vi "fill the pulse memory_12 memors.vi"(10 "memory units":T1={"Memory In"="pulse on memory", "Memory In 2"="", "Memory In 3"="", "Memory In 6"="pulse on memory", "Memory In 4"="pulse on memory", "Memory In 5"="", "Memory In 7"="", "Memory In 8"="pulse on memory", "Memory In 9"="pulse on memory", "Memory In 10"="", "Memory In 11"="", "Memory In 12"="pulse on memory"}, 11 "FIFO In":refnum<k21>="fifo pulse from host") -> ()   [LabVIEW 2021]
uses:
  <vilib>/rvi/DataTransferAndStorage/Container/Common/niFpgaContainerExecOnDevCompGetState.vi
  <vilib>/rvi/Emulation/niFpgaEmulationIsFPGAContextNoSignature.vi
  <vilib>/rvi/DataTransferAndStorage/Container/Common/niFpgaContainerGetUniqueNameForEmu.vi
  <vilib>/rvi/Emulation/niFpgaProcessEmulError.vi
  <vilib>/rvi/Emulation/niFpgaSctlEmulationGetInTimedLoop.vi
  <vilib>/rvi/errors/nirviReportUnexpectedCaseInternalError (U32).vi
  <vilib>/rvi/Memory/Memory_Emulation/niFpgaMemoryEmulationCacheClearOnFirstRun.vi
  <vilib>/rvi/Memory/Memory_Emulation/nirvimemoryEmulationManagerCache_MakeExclusive.vi
  <vilib>/rvi/Memory/Memory_Emulation/niFpgaMemoryEmulationValidateCache.vi
  <vilib>/rvi/Memory/Memory_Emulation/nirvimemoryEmulationManagerCache_InsertValue.vi
  <vilib>/Utility/error.llb/Clear Errors.vi
  <vilib>/rvi/Memory/Memory_Emulation/nirvimemoryEmulationManagerCache_ReleaseExclusive.vi
  <vilib>/rvi/Memory/Memory_Emulation/nirvimemoryEmulationManagerCache_GetValue.vi
  <vilib>/rvi/Memory/Memory_Emulation/nirvimemoryEmulationManagerCache_SetValue.vi
  <vilib>/rvi/Emulation/niFpgaSctlEmulationResourceMgr.vi
  <vilib>/rvi/errors/niFpgaSetErrorForExecOnDevCompSimple.vi
  <vilib>/rvi/eio/common/nirviEmuReportErrorAndStop.vi
  <vilib>/rvi/FIFO/Fifo_Resource/nirvififoEmulationSetSize.vi
  <vilib>/rvi/FIFO/Fifo_Resource/nirviFifoEmulationQueueMgr.vi
  <instcachedir>/0/nirviFifoEmulationQueueMgr_E5CAEC123FF24DC58D834DCA3CDAA9B5.lvgen/nirviFifoEmulationQueueMgr_E5CAEC123FF24DC58D834DCA3CDAA9B5_008.vi
  <vilib>/rvi/FIFO/Fifo_Resource/nirvififoEmulationDetermineInputValidOut.vi
  <vilib>/rvi/FIFO/Fifo_Resource/nirvififoEmulationCreateLock.vi
  <vilib>/rvi/FIFO/Fifo_Resource/nirvififoEmulationObtainLock.vi
  <vilib>/rvi/FIFO/Fifo_Resource/nirvififoEmulationReleaseLock.vi
  <vilib>/rvi/occurrence/nirviWaitOnOccurrenceBase.vi
  <vilib>/rvi/errors/nirviReportUnexpectedCaseInternalError.vi
  <vilib>/rvi/interface/RandomDataEmulation/niFpgaRandomDataHandleErrors.vi
  <vilib>/rvi/DataTransferAndStorage/Container/XNode/niFpgaContainer.xnode
  <vilib>/rvi/Memory/Memory_Emulation/niFpgaMemoryEmulationRefIn.vi
  <vilib>/rvi/FIFO/Fifo_Resource/niFpgaFifoEmulationRefIn.vi
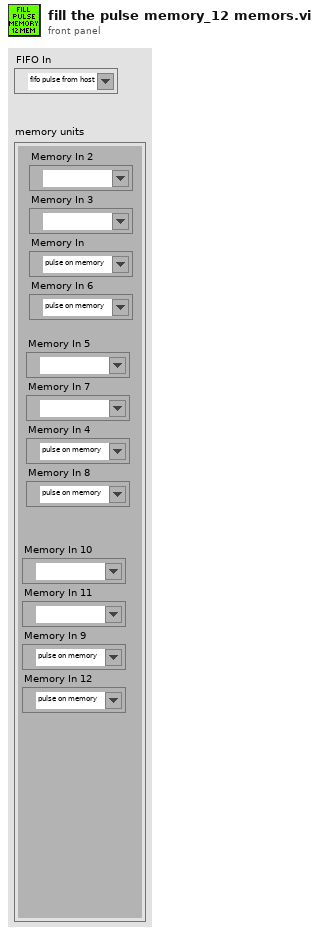
[diagram p1: front panel]
types:
  T1 = cluster{"Memory In":refnum<k21>, "Memory In 2":refnum<k21>, "Memory In 3":refnum<k21>, "Memory In 6":refnum<k21>, "Memory In 4":refnum<k21>, "Memory In 5":refnum<k21>, "Memory In 7":refnum<k21>, "Memory In 8":refnum<k21>, "Memory In 9":refnum<k21>, "Memory In 10":refnum<k21>, "Memory In 11":refnum<k21>, "Memory In 12":refnum<k21>}
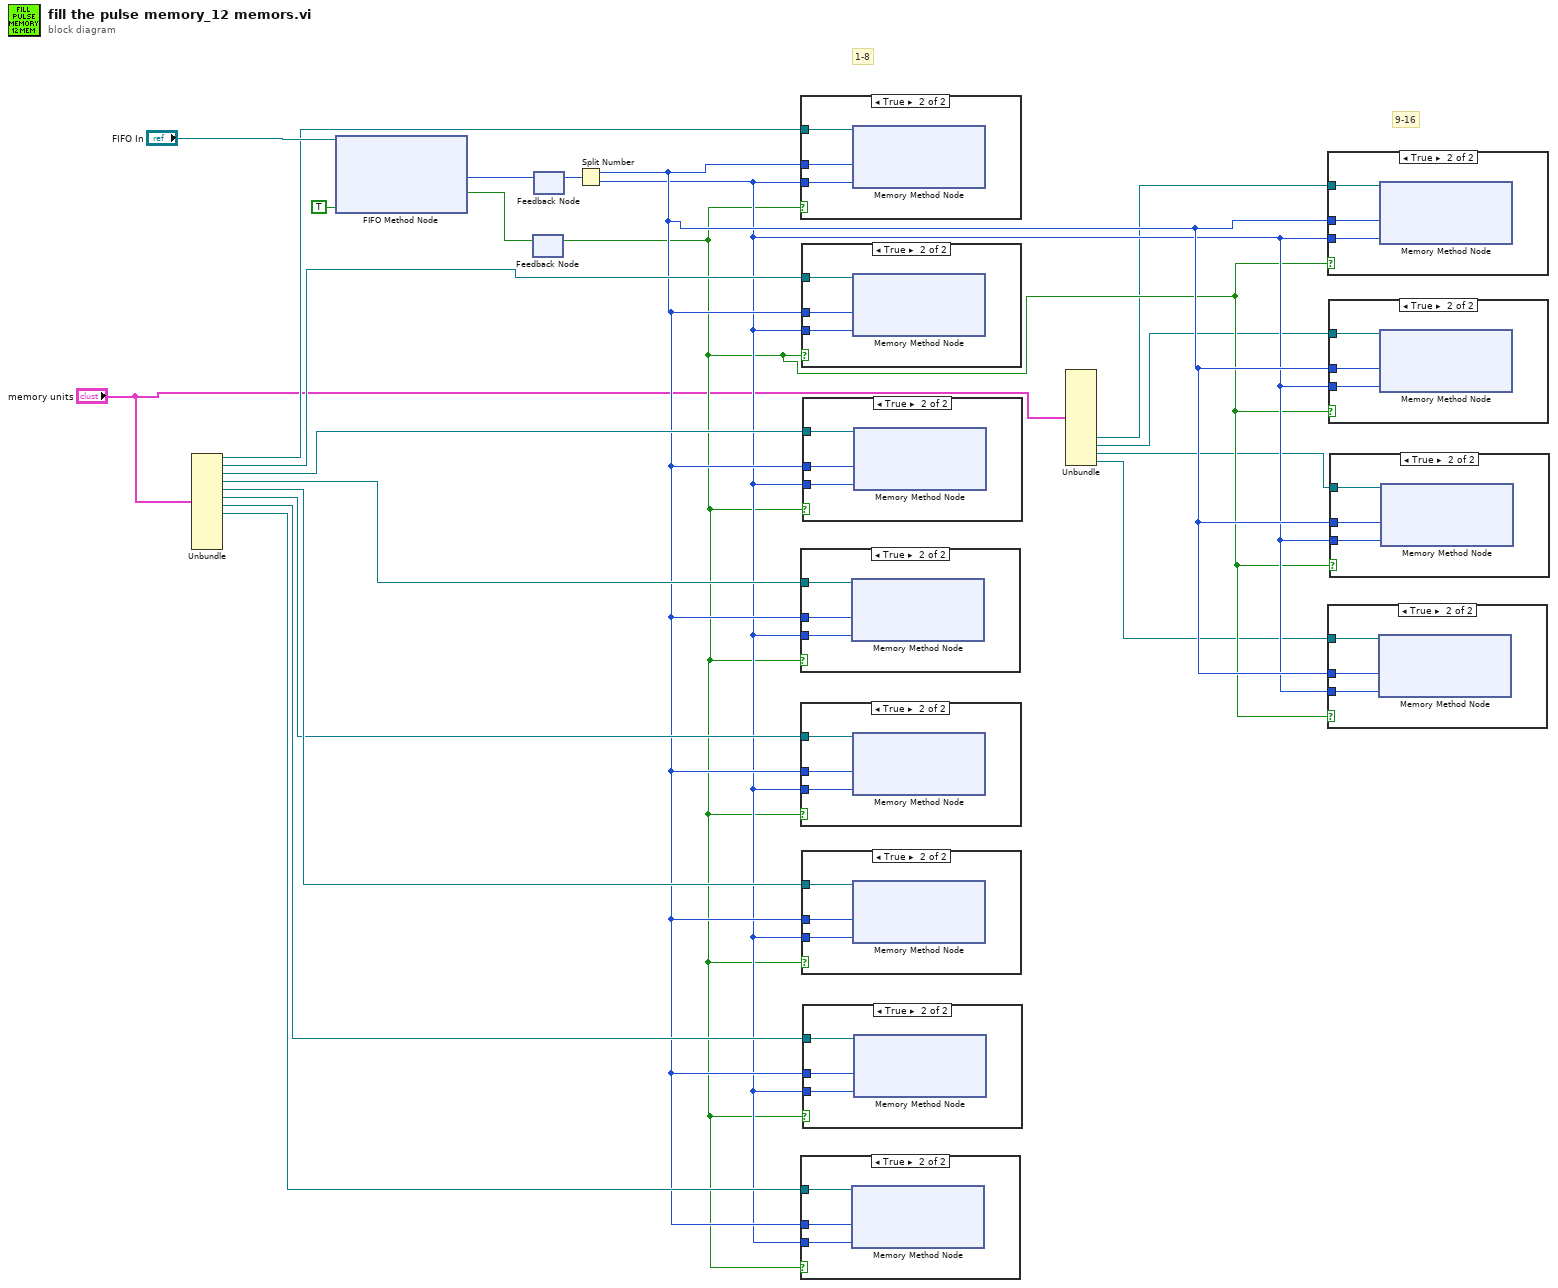
[diagram p0: block diagram]
diagram:
  # "9-16"
  # "1-8"
  n1 = Unbundle("memory units") -> ("Memory In"=w19:refnum<k21>, "Memory In 2"=w18:refnum<k21>, "Memory In 3"=w17:refnum<k21>, "Memory In 6"=w16:refnum<k21>, "Memory In 4"=w15:refnum<k21>, "Memory In 5"=w14:refnum<k21>, "Memory In 7"=w13:refnum<k21>, "Memory In 8"=w12:refnum<k21>)  [unwired: 4 out]
  n2 = xnode ("FIFO Method Node")("Ready for Output"=TRUE, "FIFO In"="FIFO In") -> ("Element"=w10:u64, "Output Valid"=w11:bool)  [unwired: 1 out]
  n3 = feedback-in #1(w11) -> ()
  n4 = feedback #1() -> (w6:bool)  [unwired: 1 in]
  n5 = feedback #2() -> (w9:u64)  [unwired: 1 in]
  n6 = feedback-in #2(w10) -> ()
  n7 = Split Number(x=w9) -> (hi(x)=w8:u32, lo(x)=w7:u32)
  n8 = case shown="True" w6 {
    tunnel: w8 -> [_ w24]
    tunnel: w7 -> [_ w23]
    tunnel: w19 -> [_ w22]
    frame False {
    }
    frame True {
      n9 = xnode ("Memory Method Node")("Address"=w24, "Data"=w23, "Memory In"=w22) -> ()  [unwired: 1 out]
    }
  }
  n10 = case shown="True" w6 {
    tunnel: w8 -> [_ w27]
    tunnel: w7 -> [_ w26]
    tunnel: w16 -> [_ w25]
    frame False {
    }
    frame True {
      n11 = xnode ("Memory Method Node")("Address"=w27, "Data"=w26, "Memory In"=w25) -> ()  [unwired: 1 out]
    }
  }
  n12 = case shown="True" w6 {
    tunnel: w8 -> [_ w30]
    tunnel: w7 -> [_ w29]
    tunnel: w14 -> [_ w28]
    frame False {
    }
    frame True {
      n13 = xnode ("Memory Method Node")("Address"=w30, "Data"=w29, "Memory In"=w28) -> ()  [unwired: 1 out]
    }
  }
  n14 = case shown="True" w6 {
    tunnel: w8 -> [_ w33]
    tunnel: w7 -> [_ w32]
    tunnel: w12 -> [_ w31]
    frame False {
    }
    frame True {
      n15 = xnode ("Memory Method Node")("Address"=w33, "Data"=w32, "Memory In"=w31) -> ()  [unwired: 1 out]
    }
  }
  n16 = case shown="True" w6 {
    tunnel: w8 -> [_ w36]
    tunnel: w7 -> [_ w35]
    tunnel: w18 -> [_ w34]
    frame False {
    }
    frame True {
      n17 = xnode ("Memory Method Node")("Address"=w36, "Data"=w35, "Memory In"=w34) -> ()  [unwired: 1 out]
    }
  }
  n18 = case shown="True" w6 {
    tunnel: w8 -> [_ w39]
    tunnel: w7 -> [_ w38]
    tunnel: w15 -> [_ w37]
    frame False {
    }
    frame True {
      n19 = xnode ("Memory Method Node")("Address"=w39, "Data"=w38, "Memory In"=w37) -> ()  [unwired: 1 out]
    }
  }
  n20 = case shown="True" w6 {
    tunnel: w8 -> [_ w42]
    tunnel: w7 -> [_ w41]
    tunnel: w17 -> [_ w40]
    frame False {
    }
    frame True {
      n21 = xnode ("Memory Method Node")("Address"=w42, "Data"=w41, "Memory In"=w40) -> ()  [unwired: 1 out]
    }
  }
  n22 = case shown="True" w6 {
    tunnel: w8 -> [_ w45]
    tunnel: w7 -> [_ w44]
    tunnel: w13 -> [_ w43]
    frame False {
    }
    frame True {
      n23 = xnode ("Memory Method Node")("Address"=w45, "Data"=w44, "Memory In"=w43) -> ()  [unwired: 1 out]
    }
  }
  n24 = Unbundle("memory units") -> ("Memory In 9"=w1:refnum<k21>, "Memory In 10"=w2:refnum<k21>, "Memory In 11"=w3:refnum<k21>, "Memory In 12"=w4:refnum<k21>)  [unwired: 8 out]
  n25 = case shown="True" w6 {
    tunnel: w8 -> [_ w48]
    tunnel: w7 -> [_ w47]
    tunnel: w1 -> [_ w46]
    frame False {
    }
    frame True {
      n26 = xnode ("Memory Method Node")("Address"=w48, "Data"=w47, "Memory In"=w46) -> ()  [unwired: 1 out]
    }
  }
  n27 = case shown="True" w6 {
    tunnel: w8 -> [_ w51]
    tunnel: w7 -> [_ w50]
    tunnel: w4 -> [_ w49]
    frame False {
    }
    frame True {
      n28 = xnode ("Memory Method Node")("Address"=w51, "Data"=w50, "Memory In"=w49) -> ()  [unwired: 1 out]
    }
  }
  n29 = case shown="True" w6 {
    tunnel: w8 -> [_ w54]
    tunnel: w7 -> [_ w53]
    tunnel: w2 -> [_ w52]
    frame False {
    }
    frame True {
      n30 = xnode ("Memory Method Node")("Address"=w54, "Data"=w53, "Memory In"=w52) -> ()  [unwired: 1 out]
    }
  }
  n31 = case shown="True" w6 {
    tunnel: w8 -> [_ w57]
    tunnel: w7 -> [_ w56]
    tunnel: w3 -> [_ w55]
    frame False {
    }
    frame True {
      n32 = xnode ("Memory Method Node")("Address"=w57, "Data"=w56, "Memory In"=w55) -> ()  [unwired: 1 out]
    }
  }
